vi "Configure Relative Measurement Level.vi"(0 "VISA resource name":refnum<visa-resource-name>, 1 "Resistance Level (0 Ohm)":dbl, 2 "Power Level (0 W)":dbl, 5 "Source Measure Unit Channel (0: Channel A)":i32(ring) items=["Channel A", "Channel B"], 7 "Measurement Function (0: Current)":i32(ring) items=["Current", "Voltage", "Resistance", "Power"], 9 "Current Level (0 A)":dbl, 11 "error in (no error)":errorcluster, 12 "Voltage Level (0 V)":dbl) -> (4 "VISA resource name out":refnum<visa-resource-name>, 15 "error out":errorcluster)   [LabVIEW 2019, in "Keithley 2600 Series.lvlib"]
doc: "Configures the offset value for relative measurements. \n\n<b>Note:</b>\nWhen the relative measurements is enabled by <b>Enable Relative Measurement</b> VI, each returned measured relative reading will be the result of the following calculation: Relative reading = Actual measured reading - Relative offset value."
uses:
  Keithley 2600 Series.lvlib
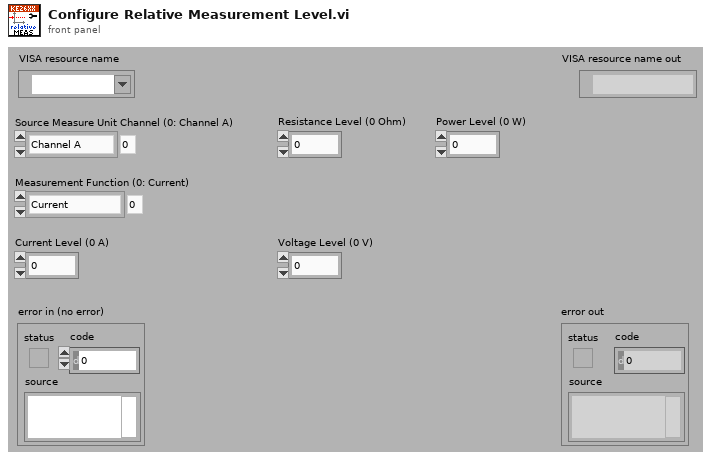
[diagram p1: front panel]
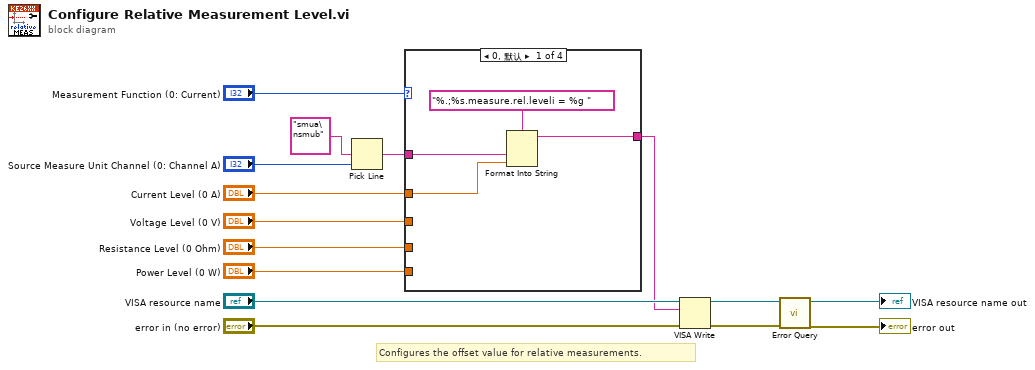
[diagram p0: block diagram]
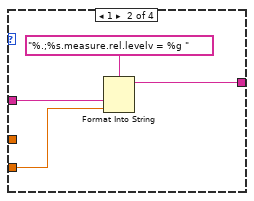
[diagram p2: hidden frame]
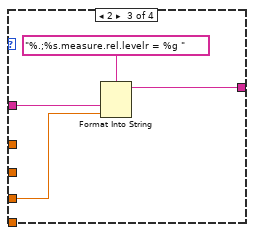
[diagram p3: hidden frame]
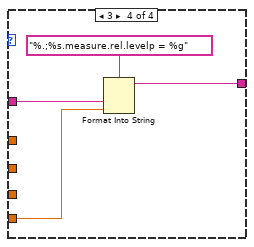
[diagram p4: hidden frame]
diagram:
  # "Configures the offset value for relative measurements."
  n1 = Pick Line(multi-line string="smua\nsmub", line index="Source Measure Unit Channel (0: Channel A)") -> (output string=w7:string)  [unwired: 1 in]
  n2 = case shown="0, 默认" "Measurement Function (0: Current)" {
    tunnel: w7 -> [w18 w22 w25 w29]
    tunnel: "Voltage Level (0 V)" -> [_ w21 _ _]
    tunnel: "Current Level (0 A)" -> [w17 _ _ _]
    tunnel: "Resistance Level (0 Ohm)" -> [_ _ w24 _]
    tunnel: "Power Level (0 W)" -> [_ _ _ w30]
    tunnel: [w16 w20 w26 w28] -> w1
    frame 0, Default {
      n3 = Format Into String(format string="%.;%s.measure.rel.leveli = %g ", w18, w17) -> (resulting string=w16:string)  [unwired: 2 in, 1 out]
    }
    frame 1 {
      n4 = Format Into String(format string="%.;%s.measure.rel.levelv = %g ", w22, w21) -> (resulting string=w20:string)  [unwired: 2 in, 1 out]
    }
    frame 2 {
      n5 = Format Into String(format string="%.;%s.measure.rel.levelr = %g ", w25, w24) -> (resulting string=w26:string)  [unwired: 2 in, 1 out]
    }
    frame 3 {
      n6 = Format Into String(format string="%.;%s.measure.rel.levelp = %g", w29, w30) -> (resulting string=w28:string)  [unwired: 2 in, 1 out]
    }
  }
  n7 = VISA Write(VISA resource name="VISA resource name", write buffer=w1, error in (no error)="error in (no error)") -> (VISA resource name out=w13:refnum<visa-resource-name>, error out=w12:errorcluster)  [unwired: 1 out]
  n8 = call "Error Query.vi"("error in (no error)"=w12, "VISA resource name"=w13) -> ("error out"=→"error out":errorcluster, "VISA resource name out"=→"VISA resource name out":refnum<visa-resource-name>)  [unwired: 6 in, 2 out]
